vi "start.vi"(8 "error in (no error)":errorcluster, 11 "WriteSignalsDAQmxPlugin in":refnum<class "SignalWriterDL090202DAQmx.lvclass">) -> (0 "error out":errorcluster, 3 "WriteSignalsDAQmxPlugin out":refnum<class "SignalWriterDL090202DAQmx.lvclass">)   [LabVIEW 2010, in "SignalWriterDL090202DAQmx.lvclass"]
uses:
  SignalWriterDL090202DAQmx.lvclass
  C:/Program Files (x86)/National Instruments/LabVIEW 2010/resource/objmgr/daqmx.rc
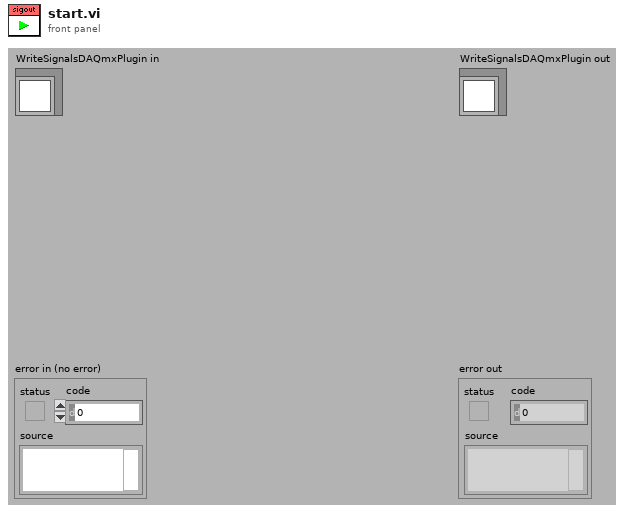
[diagram p1: front panel]
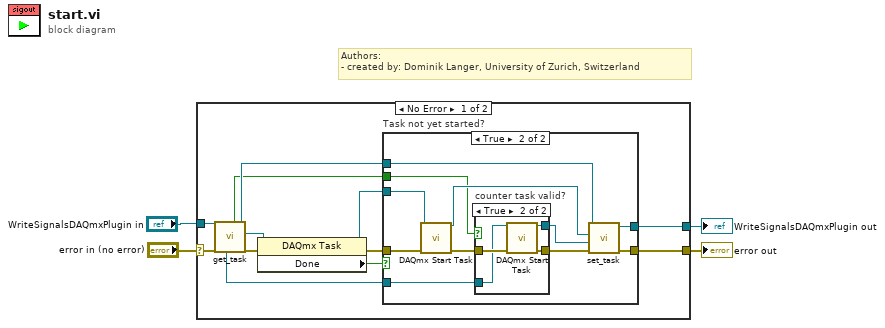
[diagram p0: block diagram]
diagram:
  # "Authors: \n- created by: Dominik Langer, University of Zurich, Switzerland"
  n1 = case shown="No Error" "error in (no error)" {
    selector: "error in (no error)" -> [w16 w37]
    tunnel: [w14 w37] -> w3
    tunnel: [w12 w36] -> w1
    tunnel: "WriteSignalsDAQmxPlugin in" -> [w15 w36]
    frame No Error {
      n2 = call-dynamic "get_task.vi"("error in (no error)"=w16, "DAQmxWriteSignals in"=w15) -> ("error out"=w11:errorcluster, "writer task"=w9:refnum<k21>, "DAQmxWriteSignals out"=w13:refnum<class "SignalWriterDL090202DAQmx.lvclass">, "counter task valid?"=w5:bool, "counter task"=w6:refnum<k21>)  [unwired: 5 out]
      n3 = property class="DAQmx Task"(reference=w9, error in=w11) -> (reference out=w8:refnum<k21>, error out=w10:errorcluster, "Done"=w7:bool)
      n4 = case "Task not yet started?" shown="True" w7 {
        tunnel: [w17 w29] -> w14
        tunnel: w13 -> [w18 w24]
        tunnel: [w18 w28] -> w12
        tunnel: w10 -> [w17 w25]
        tunnel: w8 -> [_ w26]
        tunnel: w6 -> [_ w21]
        tunnel: w5 -> [_ w19]
        frame False {
        }
        frame True {
          n5 = call <vilib>:"DAQmx Start Task.vi"("task/channels in"=w26, "error in"=w25) -> ("task out"=w27:refnum<k21>, "error out"=w23:errorcluster)  [unwired: 12 out]
          n6 = case "counter task valid?" shown="True" w19 {
            tunnel: w23 -> [w30 w35]
            tunnel: [w30 w34] -> w22
            tunnel: w21 -> [w31 w33]
            tunnel: [w31 w32] -> w20
            frame False {
            }
            frame True {
              n7 = call <vilib>:"DAQmx Start Task.vi"("task/channels in"=w33, "error in"=w35) -> ("task out"=w32:refnum<k21>, "error out"=w34:errorcluster)  [unwired: 12 out]
            }
          }
          n8 = call-dynamic "set_task.vi"("error in (no error)"=w22, "counter task"=w20, "output task"=w27, "DAQmxWriteSignals in"=w24) -> ("error out"=w29:errorcluster, "DAQmxWriteSignals out"=w28:refnum<class "SignalWriterDL090202DAQmx.lvclass">)  [unwired: 6 out]
        }
      }
    }
    frame Error {
    }
  }
  "error out" <- w3
  "WriteSignalsDAQmxPlugin out" <- w1
